vi "Copy Data Files to Server.vi"(11 "Error In":errorcluster) -> (15 "Error Out":errorcluster)   [LabVIEW 2013]
uses:
  <vilib>/Utility/config.llb/Read Key (Path).vi
  <vilib>/Utility/config.llb/Read Key (String).vi
  <vilib>/Utility/config.llb/Read Key (Boolean).vi
  <vilib>/Utility/config.llb/NI_LVConfig.lvlib
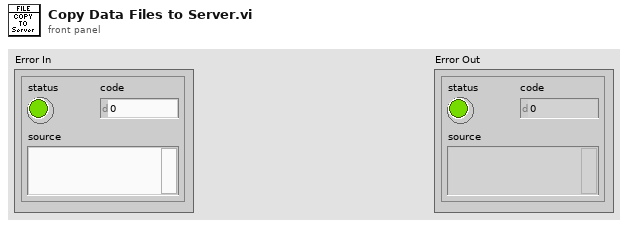
[diagram p1: front panel]
types:
  T1 = typedef "NI_LVConfig.lvlib/Config Data RefNum.ctl" = refnum<k1>
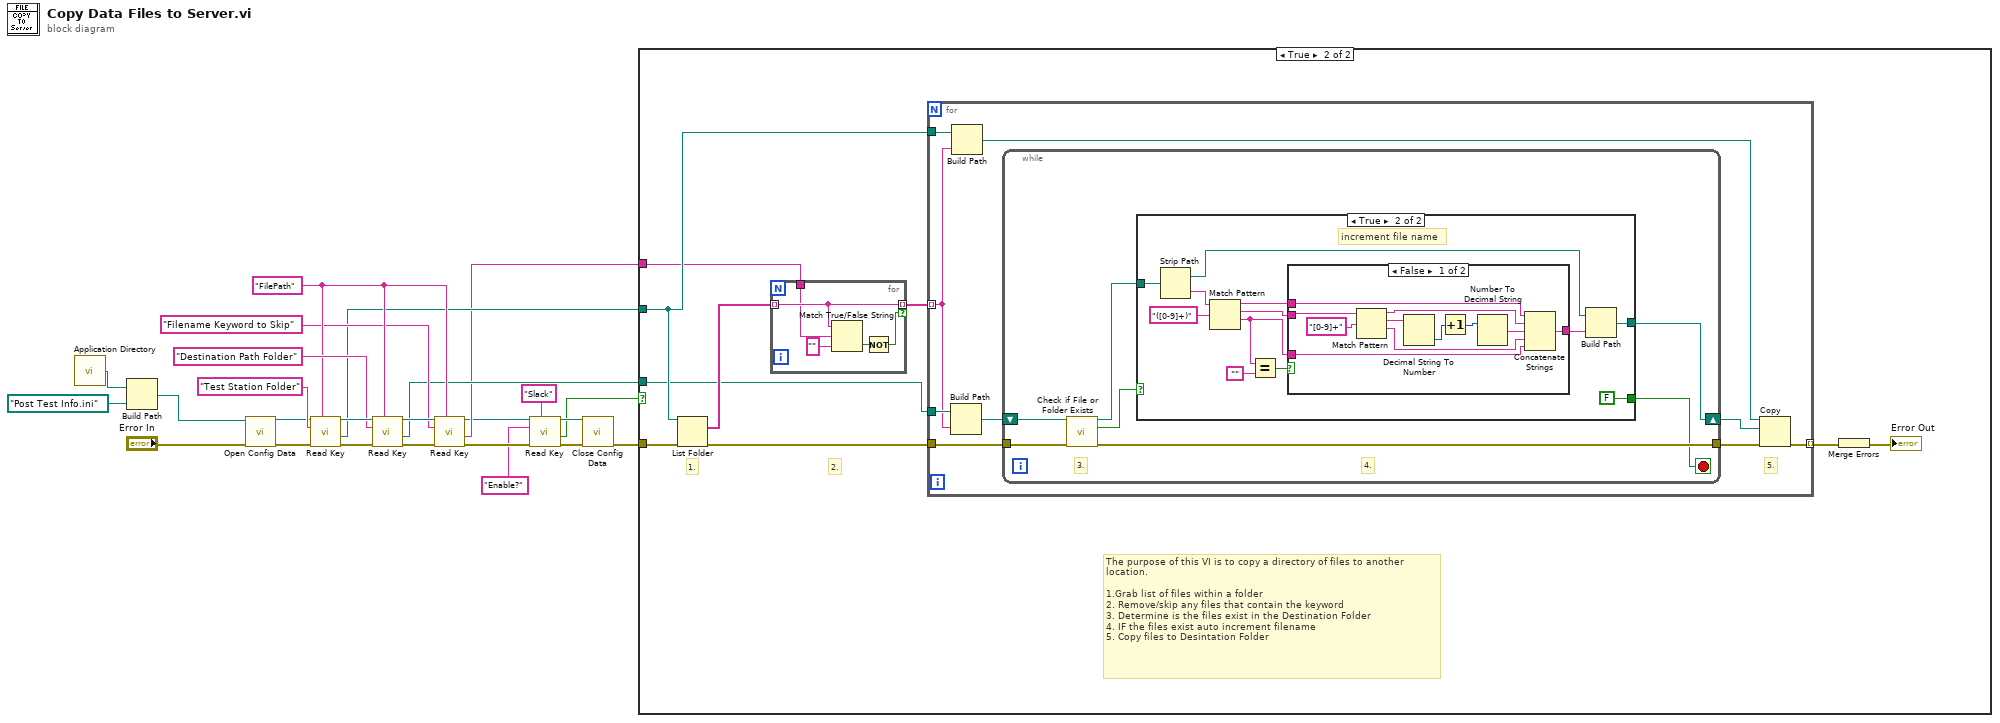
[diagram p0: block diagram]
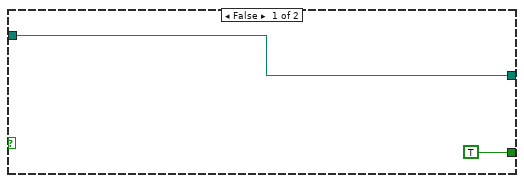
[diagram p3: hidden frame]
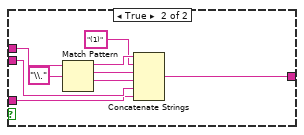
[diagram p4: hidden frame]
diagram:
  w19 = "FilePath" ("section")
  n1 = call <vilib>:"Application Directory.vi"() -> ("Application Directory"=w10:path)
  n2 = Build Path(base path=w10, name or relative path=path "Post Test Info.ini" ("default name")) -> (appended path=w1:path)
  n3 = call <vilib>:"Open Config Data.vi"("error in (no error)"="Error In", "configuration file path"=w1) -> ("error out"=w16:errorcluster, "refnum"=w17:T1)  [unwired: 7 in, 1 out]
  n4 = call-poly <vilib>:"Read Key.vi"("section"=w19, "error in (no error)"=w16, "key"="Test Station Folder", "refnum"=w17) -> ("error out"=w24:errorcluster, "value"=w15:path, "refnum out"=w23:T1)  [unwired: 4 in, 1 out]
  n5 = call-poly <vilib>:"Read Key.vi"("section"=w19, "error in (no error)"=w24, "key"="Destination Path Folder", "refnum"=w23) -> ("error out"=w20:errorcluster, "value"=w14:path, "refnum out"=w21:T1)  [unwired: 4 in, 1 out]
  n6 = call-poly <vilib>:"Read Key.vi"("section"=w19, "error in (no error)"=w20, "key"="Filename Keyword to Skip", "refnum"=w21) -> ("error out"=w8:errorcluster, "value"=w13:string, "refnum out"=w6:T1)  [unwired: 4 in, 1 out]
  n7 = call-poly <vilib>:"Read Key.vi"("section"="Slack", "error in (no error)"=w8, "key"="Enable?", "refnum"=w6) -> ("error out"=w7:errorcluster, "value"=w2:bool, "refnum out"=w5:T1)  [unwired: 4 in, 1 out]
  n8 = call <vilib>:"Close Config Data.vi"("error in (no error)"=w7, "refnum"=w5) -> ("error out"=w12:errorcluster)  [unwired: 8 in, 1 out]
  n9 = case shown="True" w2 {
    tunnel: w15 -> [_ w29]
    tunnel: w14 -> [_ w28]
    tunnel: w13 -> [_ w27]
    tunnel: w12 -> [_ w26]
    frame False {
    }
    frame True {
      # "2."
      # "1."
      # "The purpose of this VI is to copy a directory of files to another location.\n\n1.Grab list of files within a folder\n2. Remove/skip any files that contain the keyword\n3. Determine is the files exist in the Destination Folder\n4. IF the files exist auto increment filename\n5. Copy files to Desintation Folder"
      n10 = List Folder(path=w29, error in=w26) -> (filenames=w34:string[], error out=w30:errorcluster)  [unwired: 2 in, 2 out]
      n11 = for {
        tunnel: w34 -> [w89] mode=indexing
        tunnel: [w89] -> w33 mode=indexing if=w87
        tunnel: w27 -> [w85]
        n12 = Match True/False String(2:"" ("false string"), 3:w85, 4:w89) -> (0:w86:bool)  [unwired: 1 out]
        n13 = Not(x=w86) -> (.not. x?=w87:bool)
      }
      n14 = for {
        tunnel: w29 -> [w43]
        tunnel: w33 -> [w40] mode=indexing
        tunnel: w28 -> [w41]
        tunnel: [w38] -> w32 mode=indexing
        tunnel: w30 -> [w37]
        # "5."
        n15 = Build Path(base path=w41, name or relative path=w40) -> (appended path=w36:path)
        n16 = Build Path(base path=w43, name or relative path=w40) -> (appended path=w42:path)
        n17 = while {
          tunnel: [w48] -> w39
          tunnel: w37 -> [w47]
          shift-right: [w44] -> w35
          shift-left: w36 -> [w45]
          stop <- w46 stop-if-true
          # "4."
          # "3."
          n18 = call <vilib>:"Check if File or Folder Exists.vi"("error in (no error)"=w47, "path"=w45) -> ("error out"=w48:errorcluster, "file or folder exists?"=w50:bool, "dup path"=w49:path)  [unwired: 7 in]
          n19 = case shown="True" w50 {
            tunnel: [w52 w59] -> w44
            tunnel: w49 -> [w52 w54]
            tunnel: [TRUE FALSE] -> w46
            frame False {
            }
            frame True {
              # "increment file name"
              n20 = Strip Path(path=w54) -> (stripped path=w58:path, name=w64:string)
              n21 = Match Pattern(string=w64, regular expression="([0-9]+)") -> (before substring=w60:string, match substring=w56:string, after substring=w55:string)  [unwired: 1 in, 1 out]
              n22 = Equal?(x=w55, y="") -> (x = y?=w61:bool)
              n23 = case shown="False" w61 {
                tunnel: w60 -> [w65 w84]
                tunnel: [w69 w76] -> w57
                tunnel: w56 -> [w75 w78]
                tunnel: w55 -> [w66 w77]
                frame False {
                  n24 = Match Pattern(string=w75, regular expression="[0-9]+") -> (before substring=w68:string, match substring=w73:string, after substring=w67:string)  [unwired: 1 in, 1 out]
                  n25 = Decimal String To Number(string=w73) -> (number=w72:i32)  [unwired: 2 in, 1 out]
                  n26 = Increment(x=w72) -> (x+1=w71:i32)
                  n27 = Number To Decimal String(number=w71) -> (decimal integer string=w70:string)  [unwired: 1 in]
                  n28 = Concatenate Strings(w65, w68, w70, w67, w66) -> (w69:string)
                }
                frame True {
                  n29 = Match Pattern(string=w84, regular expression="\\.") -> (before substring=w82:string, match substring=w80:string, after substring=w79:string)  [unwired: 1 in, 1 out]
                  n30 = Concatenate Strings(w82, "(1)" ("string"), w80, w79, w78, w77) -> (w76:string)
                }
              }
              n31 = Build Path(base path=w58, name or relative path=w57) -> (appended path=w59:path)
            }
          }
        }
        n32 = Copy(8:w39, 10:w35, 11:w42) -> (0:w38:errorcluster)  [unwired: 2 in, 2 out]
      }
      n33 = Merge Errors(w32) -> (→"Error Out":errorcluster)
    }
  }
